vi "Actor Core.vi"(8 "error in":errorcluster, 11 "TCPIP Communications in":refnum<class "TCPIP Communications.lvclass">) -> (0 "error out":errorcluster, 3 "Actor out":refnum<class "Actor.lvclass">)   [LabVIEW 2015, in "TCPIP Communications Framework.lvlib" / "TCPIP Communications.lvclass"]
doc: "(<B>Filename</B>: Actor Framework.lvlib:Actor.lvclass:Actor Core.vi)\n\nReceives messages to the actor, reacts to them, and initiates any error handling that may shut the actor down.\n\nDescendant classes may override this VI to append parallel tasks for the actor to complete while it handles messages. Overrides use the Call Parent Method node."
uses:
  TCPIP Communications.lvclass
  <vilib>/ActorFramework/Actor/Actor.lvclass
  <vilib>/ActorFramework/Actor/Actor.lvclass/Actor.ctl
  <vilib>/ActorFramework/Message Enqueuer/Message Enqueuer.lvclass/Message Enqueuer.ctl
  TCPIP Communications.lvclass/TCPIP Communications.ctl
  <vilib>/ActorFramework/Message Enqueuer/Init from Existing Queue.vi
  <vilib>/ActorFramework/Message Enqueuer/Enqueue.vi
  <vilib>/ActorFramework/Message Priority Queue/Priority Enqueue.vi
  <vilib>/ActorFramework/Message Enqueuer/Message Enqueuer.lvclass
  TCPIP Communications Messages/Open Reception Msg/Open Reception Msg.lvclass
  TCPIP Communications Messages/Open Transmission Msg/Open Transmission Msg.lvclass
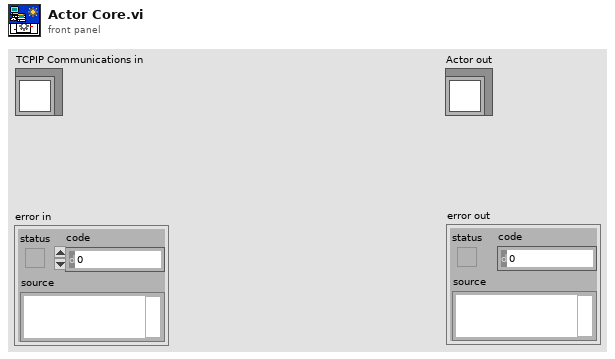
[diagram p1: front panel]
types:
  T1 = typedef "TCPIP Communications Framework.lvlib/TCPIP Communications.lvclass/Mode Select.ctl" = enum16{"Tx/Rx", "Tx", "Rx"}
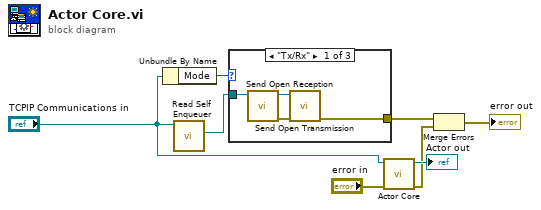
[diagram p0: block diagram]
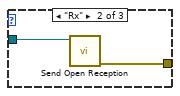
[diagram p2: hidden frame]
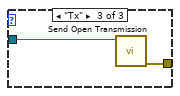
[diagram p3: hidden frame]
diagram:
  n1 = Unbundle By Name("TCPIP Communications in") -> ("Mode"=w1:T1)
  n2 = call <vilib>:"Read Self Enqueuer.vi"("Actor"="TCPIP Communications in") -> ("Self Enqueuer"=w3:refnum<class "Message Enqueuer.lvclass">)  [unwired: 10 in]
  n3 = case shown="\"Tx/Rx\"" w1 {
    tunnel: [w9 w13 w15] -> w4
    tunnel: w3 -> [w12 w14 w16]
    frame "Tx/Rx" {
      n4 = call "Send Open Reception.vi"("Message Enqueuer"=w12) -> ("error out"=w10:errorcluster, "Message Enqueuer out"=w11:refnum<class "Message Enqueuer.lvclass">)  [unwired: 9 in]
      n5 = call "Send Open Transmission.vi"("error in (no error)"=w10, "Message Enqueuer"=w11) -> ("error out"=w9:errorcluster)  [unwired: 8 in, 1 out]
    }
    frame "Rx" {
      n6 = call "Send Open Reception.vi"("Message Enqueuer"=w14) -> ("error out"=w13:errorcluster)  [unwired: 9 in, 1 out]
    }
    frame "Tx" {
      n7 = call "Send Open Transmission.vi"("Message Enqueuer"=w16) -> ("error out"=w15:errorcluster)  [unwired: 9 in, 1 out]
    }
  }
  n8 = call-parent "Actor Core.vi"("error in"="error in", "Actor in"="TCPIP Communications in") -> ("error out"=w7:errorcluster, "Actor out"=→"Actor out":refnum<class "Actor.lvclass">)  [unwired: 8 in]
  n9 = Merge Errors(w4, w7) -> (→"error out":errorcluster)
